vi "Parse Basic String.vi"(8 "error in (no error)":errorcluster, 10 "start at":i32, 11 "TOML String":string) -> (0 "error out":errorcluster, 2 "offset past match":i32, 3 "String":string)   [LabVIEW 2020, in "TOML.lvlib"]
uses:
  TOML.lvlib
  <vilib>/regexp/Match Regular Expression.xnode
  <vilib>/ErrorRing/Error Ring.xnode
panel:
  out "before match":string
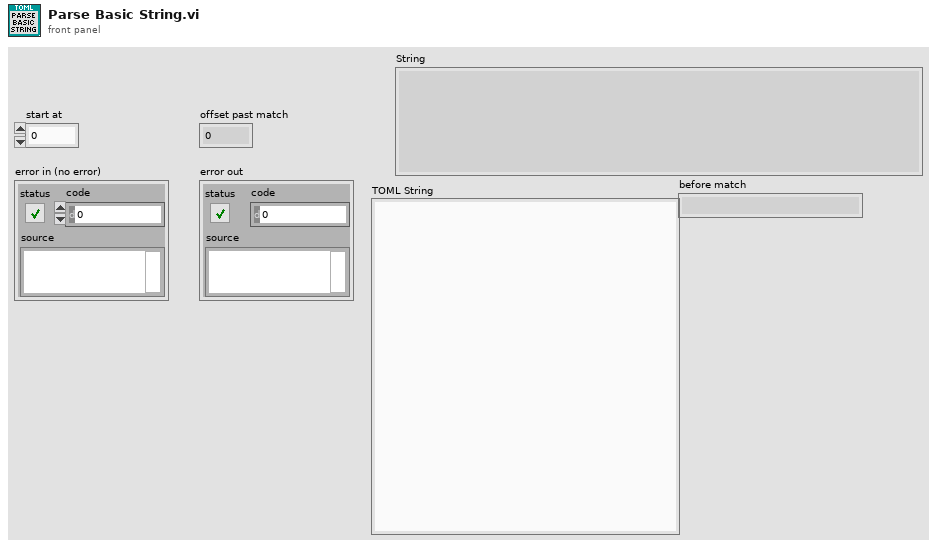
[diagram p1: front panel]
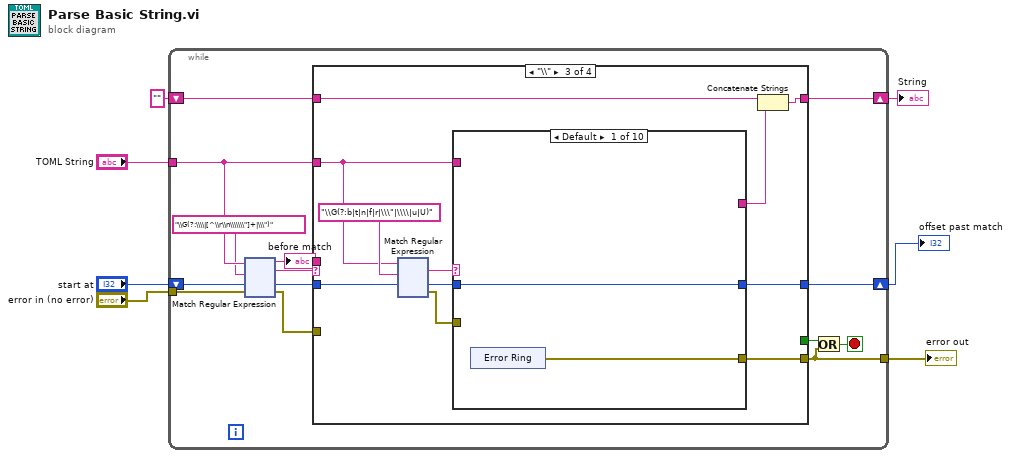
[diagram p0: block diagram]
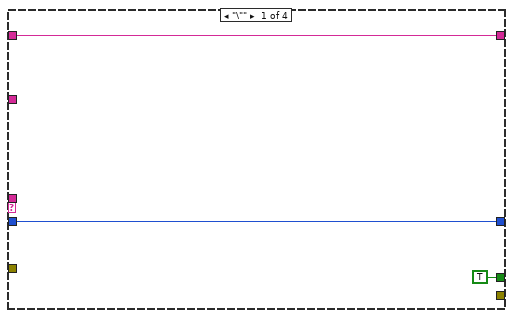
[diagram p2: hidden frame]
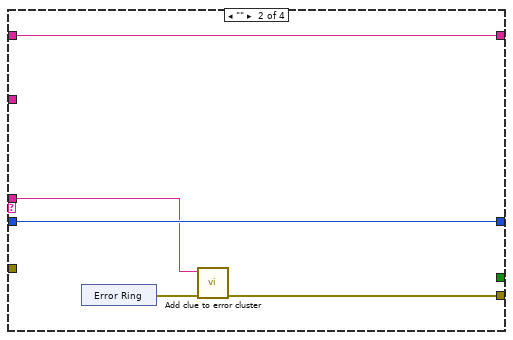
[diagram p3: hidden frame]
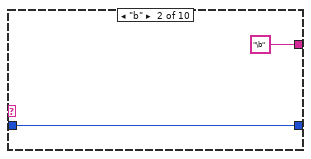
[diagram p4: hidden frame]
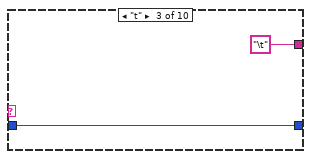
[diagram p5: hidden frame]
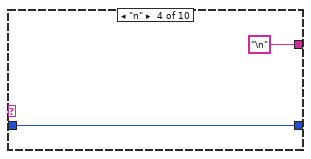
[diagram p6: hidden frame]
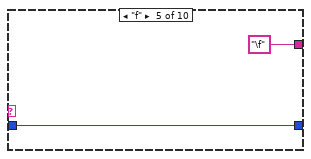
[diagram p7: hidden frame]
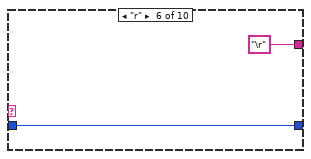
[diagram p8: hidden frame]
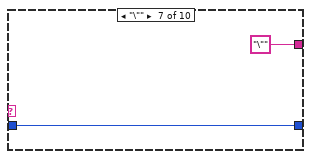
[diagram p9: hidden frame]
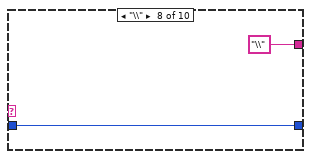
[diagram p10: hidden frame]
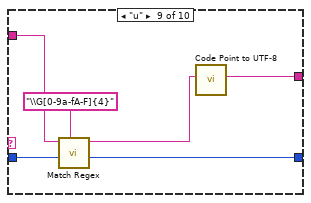
[diagram p11: hidden frame]
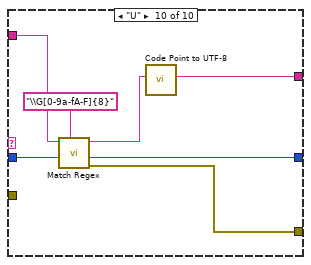
[diagram p12: hidden frame]
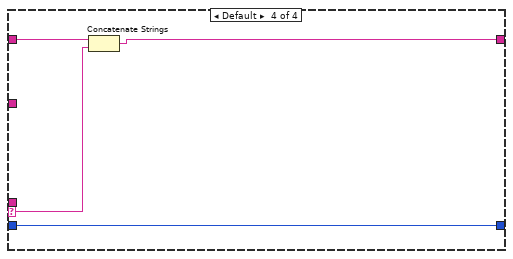
[diagram p13: hidden frame]
diagram:
  n1 = while {
    tunnel: "error in (no error)" -> [w21]
    tunnel: "TOML String" -> [w14]
    shift-right: [w19] -> w1
    shift-left: "start at" -> [w20]
    shift-right: [w17] -> w2
    shift-left: "" -> [w16]
    tunnel: [w12] -> w3
    stop <- w13 stop-if-true
    n2 = xnode "Match Regular Expression"("input string"=w14, "regular expression"="\\G(?:\\\\|[^\\r\\n\\\\\\\"]+|\\\")", "offset (0)"=w20, "error in"=w21) -> ("before match"=w8:string, "whole match"=w11:string, "offset past match"=w18:i32, "error out"=w9:errorcluster)  [unwired: 2 in, 1 out]
    "before match" <- w8
    n3 = case shown="\"\\\\\"" w11 {
      selector: w11 -> [_ _ _ w188]
      tunnel: [w23 w28 w37 w189] -> w19
      tunnel: w18 -> [w23 w28 w40 w189]
      tunnel: [w24 w29 w35 w186] -> w17
      tunnel: w16 -> [w24 w29 w41 w187]
      tunnel: [TRUE _ _ _] -> w15
      tunnel: w14 -> [_ _ w33 _]
      tunnel: [_ w26 w38 _] -> w12
      tunnel: w9 -> [_ _ _ _]
      tunnel: w8 -> [_ w25 _ _]
      frame "\"" {
      }
      frame "" {
        n4 = xnode "Error Ring"() -> ("error out"=w27:errorcluster)
        n5 = call "Add clue to error cluster.vi"("error in (no error)"=w27, "String"=w25) -> ("error out"=w26:errorcluster)  [unwired: 9 in]
      }
      frame "\\" {
        n6 = xnode "Match Regular Expression"("input string"=w33, "regular expression"="\\G(?:b|t|n|f|r|\\\"|\\\\|u|U)", "offset (0)"=w40) -> ("whole match"=w32:string, "offset past match"=w36:i32, "error out"=w31:errorcluster)  [unwired: 3 in, 2 out]
        n7 = case shown="Default" w32 {
          tunnel: [w42 _ _ _ _ _ _ _ _ w67] -> w38
          tunnel: [w43 w45 w47 w49 w51 w53 w55 w57 w61 w68] -> w37
          tunnel: w36 -> [w43 w45 w47 w49 w51 w53 w55 w57 w62 w69]
          tunnel: [_ "\b" ("regular expression") "\t" ("regular expression") "\n" ("regular expression") "\f" ("regular expression") "\r" ("regular expression") "\"" ("regular expression") "\\" ("regular expression") w59 w65] -> w34
          tunnel: w33 -> [_ _ _ _ _ _ _ _ w63 w70]
          tunnel: w31 -> [_ _ _ _ _ _ _ _ _ _]
          frame Default {
            n8 = xnode "Error Ring"() -> ("error out"=w42:errorcluster)
          }
          frame "b" {
          }
          frame "t" {
          }
          frame "n" {
          }
          frame "f" {
          }
          frame "r" {
          }
          frame "\"" {
          }
          frame "\\" {
          }
          frame "u" {
            n9 = call "Match Regex.vi"("regular expression"="\\G[0-9a-fA-F]{4}", "offset"=w62, "String"=w63) -> ("offset past match"=w61:i32, "whole match"=w60:string)  [unwired: 5 in, 2 out]
            n10 = call "Code Point to UTF-8.vi"("Code Point"=w60) -> ("UTF-8"=w59:string)  [unwired: 10 in]
          }
          frame "U" {
            n11 = call "Match Regex.vi"("regular expression"="\\G[0-9a-fA-F]{8}", "offset"=w69, "String"=w70) -> ("error out"=w67:errorcluster, "offset past match"=w68:i32, "whole match"=w66:string)  [unwired: 5 in, 1 out]
            n12 = call "Code Point to UTF-8.vi"("Code Point"=w66) -> ("UTF-8"=w65:string)  [unwired: 10 in]
          }
        }
        n13 = Concatenate Strings(w41, w34) -> (w35:string)
      }
      frame Default {
        n14 = Concatenate Strings(w187, w188) -> (w186:string)
      }
    }
    n15 = Or(x=w15, y=w12) -> (x .or. y?=w13:bool)
  }
  "error out" <- w3
  "offset past match" <- w1
  "String" <- w2
